vi "Control_GameOverGlobal.vi"() -> ()   [LabVIEW 2018]
panel:
  in  "Player4_GameOver":bool=TRUE
  in  "Player3_GameOver":bool=TRUE
  in  "Player2_GameOver":bool=TRUE
  in  "Player1_GameOver":bool=TRUE
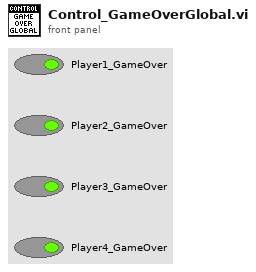
[diagram p1: front panel]
diagram:
